vi "Retrieve - Core.vi"(8 "error in (no error)":errorcluster, 10 "Error code":i32, 11 "Error Filter in":refnum<class "Error Filter.lvclass">) -> (0 "error out":errorcluster, 2 "Filter":bool, 3 "Error Filter out":refnum<class "Error Filter.lvclass">)   [LabVIEW 2026, in "TALOS.lvlib" / "Classes.lvlib" / "Error Filter.lvclass"]
uses:
  Error Filter.lvclass
  Error Filter.lvclass/Error Filter.ctl
  <vilib>/Utility/miscctls.llb/LVMapReplaceAction.ctl
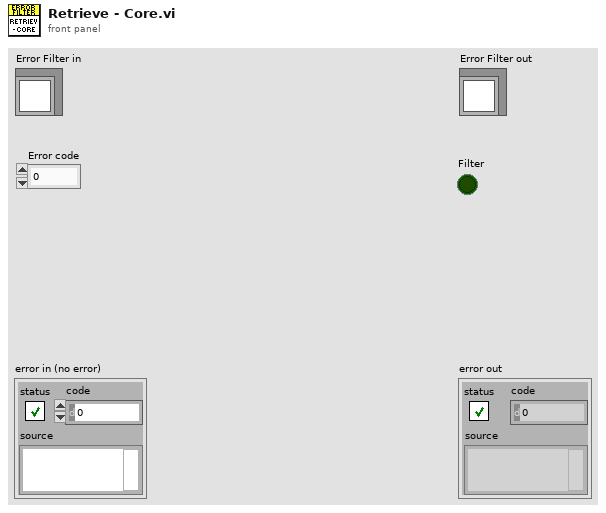
[diagram p1: front panel]
types:
  T1 = typedef "LVMapReplaceAction.ctl" = enum32{"Modify Entry only if found", "Add or Modify Entry", "Delete Entry"}
  T2 = typedef "TALOS.lvlib/Classes.lvlib/Error Filter.lvclass/Error Filter Properties.ctl" = cluster{"Repetitions":u32, "Until":timestamp}
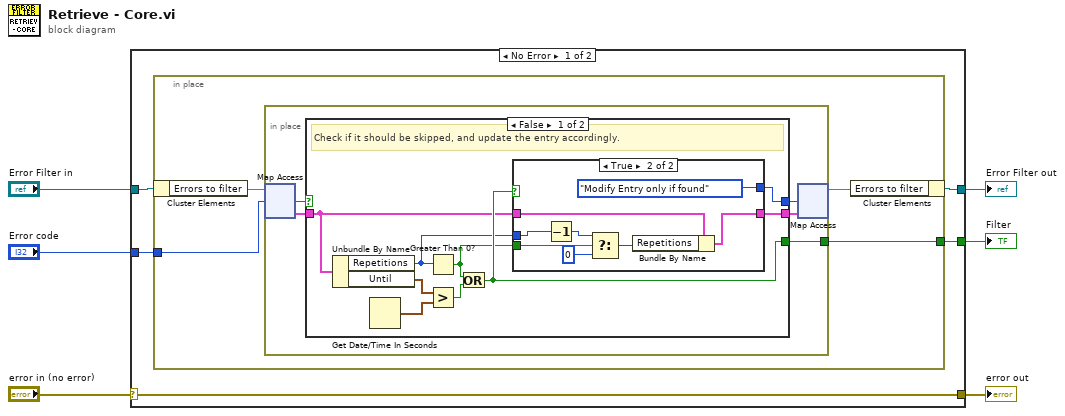
[diagram p0: block diagram]
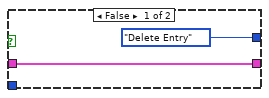
[diagram p2: hidden frame]
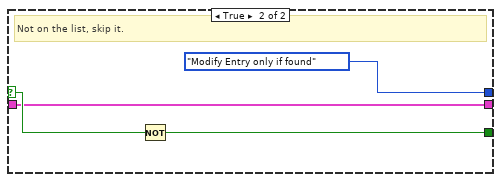
[diagram p3: hidden frame]
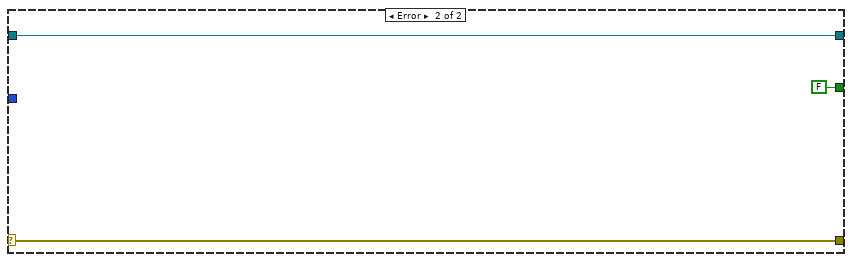
[diagram p4: hidden frame]
diagram:
  n1 = case shown="No Error" "error in (no error)" {
    selector: "error in (no error)" -> [w7 w46]
    tunnel: [w7 w46] -> w5
    tunnel: [w9 w45] -> w3
    tunnel: "Error Filter in" -> [w11 w45]
    tunnel: "Error code" -> [w10 _]
    tunnel: [w8 FALSE] -> w1
    frame No Error {
      n2 = in-place {
        in-place-border: w10 -> [w14]
        in-place-border: [w12] -> w8
        n3 = in-place-cluster #1(w11) -> ("Errors to filter"=w15:map{i32, T2})
        n4 = in-place {
          in-place-border: [w18] -> w12
          n5 = in-place-map #2(w15, w14) -> (w17:T2, w19:bool)  [unwired: 1 in]
          n6 = case shown="False" w19 {
            selector: w19 -> [_ w42]
            tunnel: [w26 LVMapReplaceAction."Modify Entry only if found" ("action")] -> w20
            tunnel: [w25 w41] -> w18
            tunnel: w17 -> [w24 w40]
            tunnel: [w22 w40] -> w16
            frame False {
              # "Check if it should be skipped, and update the entry accordingly."
              n7 = Unbundle By Name(w24) -> ("Repetitions"=w23:u32, "Until"=w29:timestamp)
              n8 = Get Date/Time In Seconds() -> (seconds since 1Jan1904=w28:timestamp)
              n9 = Greater Than 0?(x=w23) -> (x > 0?=w21:bool)
              n10 = Greater?(x=w29, y=w28) -> (0:w27:bool)
              n11 = Or(x=w21, y=w27) -> (x .or. y?=w25:bool)
              n12 = case shown="True" w25 {
                tunnel: [LVMapReplaceAction."Delete Entry" ("action") LVMapReplaceAction."Modify Entry only if found" ("action")] -> w26
                tunnel: w24 -> [w30 w39]
                tunnel: w23 -> [_ w34]
                tunnel: [w30 w38] -> w22
                tunnel: w21 -> [_ w36]
                frame False {
                }
                frame True {
                  n13 = Decrement(x=w34) -> (x-1=w33:u32)
                  n14 = Select(t=w33, s=w36, f=u32 0) -> (s? t:f=w35:u32)
                  n15 = Bundle By Name(cluster=w39, "Repetitions"=w35) -> (w38:T2)
                }
              }
            }
            frame True {
              # "Not on the list, skip it."
              n16 = Not(x=w42) -> (.not. x?=w41:bool)
            }
          }
          n17 = in-place-map #2(w16, w20) -> (w13:map{i32, T2})  [unwired: 2 out]
        }
        n18 = in-place-cluster #1("Errors to filter"=w13) -> (w9:refnum<class "Error Filter.lvclass">)
      }
    }
    frame Error {
    }
  }
  "error out" <- w5
  "Error Filter out" <- w3
  "Filter" <- w1
